vi "seconds_to_hhmmss(SubVI).vi"(0 "Total seconds":dbl) -> (4 "seconds":dbl, 6 "minutes":dbl, 10 "hours":dbl, 15 "ms":dbl)   [LabVIEW 2023]
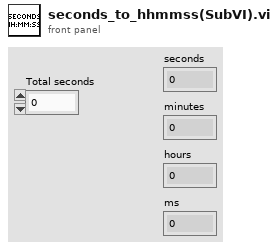
[diagram p1: front panel]
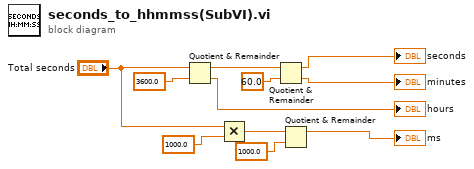
[diagram p0: block diagram]
diagram:
  n1 = Quotient & Remainder(x="Total seconds", y=3600.0) -> (x-y*floor(x/y)=w2:dbl, floor(x/y)=→"hours":dbl)
  n2 = Multiply(x="Total seconds", y=1000.0) -> (x*y=w1:dbl)
  n3 = Quotient & Remainder(x=w2, y=60.0) -> (x-y*floor(x/y)=→"seconds":dbl, floor(x/y)=→"minutes":dbl)
  n4 = Quotient & Remainder(x=w1, y=1000.0) -> (x-y*floor(x/y)=→"ms":dbl)  [unwired: 1 out]
